vi "KPI.vi"(0 "Connection In":refnum<k7>, 5 "ID compresseur":dbl, 7 "Date Debut":timestamp format="%<%.0X %x>T", 9 "Date Fin":timestamp format="%<%.0X %x>T", 11 "Error in (no error)":errorcluster) -> (1 "Temps de fonctionnement total":string, 3 "Taux d’utilisation (%)":string, 4 "Connection Out":refnum<k7>, 6 "Pression moyenne":string, 10 "température moyenne":string, 12 "Nombre de démarrages / arrêts":string, 14 "Temps d'arret total":string, 15 "Error out":errorcluster)   [LabVIEW 2019]
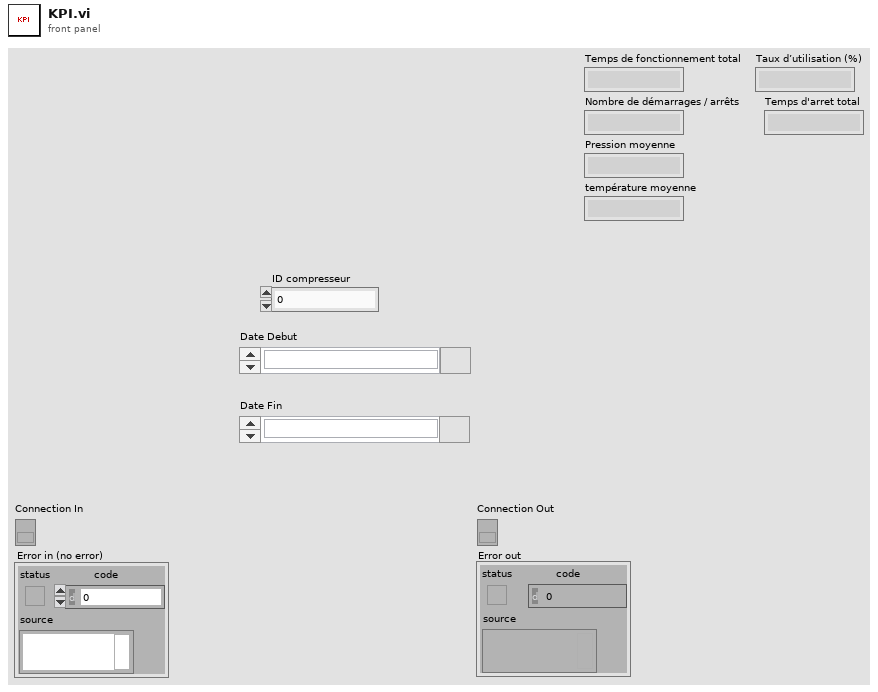
[diagram p1: front panel]
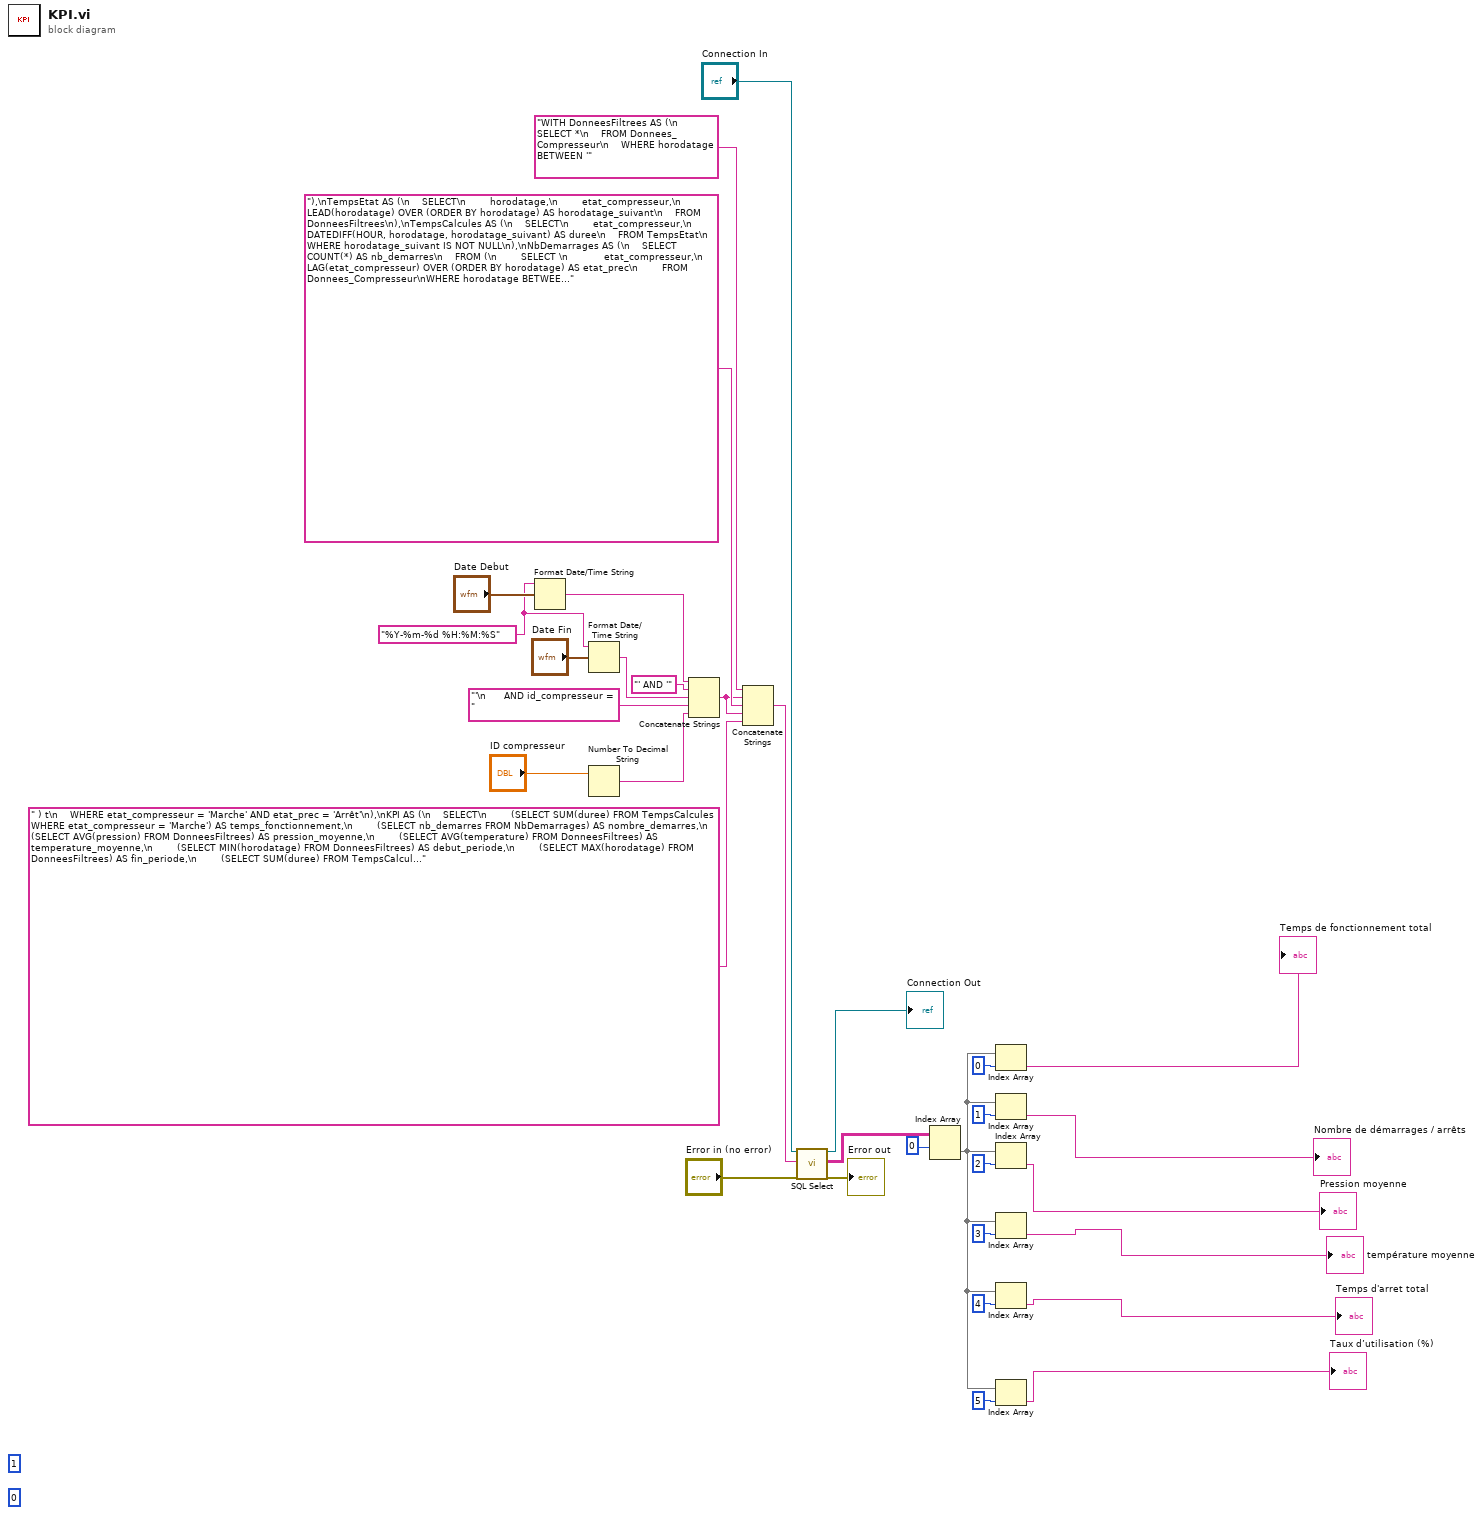
[diagram p0: block diagram]
diagram:
  (unwired) 0 ("index")
  (unwired) 1 ("index (row)")
  w29 = "%Y-%m-%d %H:%M:%S" ("time format string (%c)")
  n1 = Format Date/Time String(time format string (%c)=w29, seconds (now)="Date Debut") -> (date/time string=w25:string)  [unwired: 1 in]
  n2 = Format Date/Time String(time format string (%c)=w29, seconds (now)="Date Fin") -> (date/time string=w23:string)  [unwired: 1 in]
  n3 = Number To Decimal String(number="ID compresseur") -> (decimal integer string=w21:string)  [unwired: 1 in]
  n4 = Concatenate Strings(w25, "' AND '" ("string"), w23, "'\n      AND id_compresseur = " ("string"), w21) -> (w17:string)
  n5 = Concatenate Strings("WITH DonneesFiltrees AS (\n    SELECT *\n    FROM Donnees_Compresseur\n    WHERE horodatage BETWEEN '" ("string"), w17, "),\nTempsEtat AS (\n    SELECT\n        horodatage,\n        etat_compresseur,\n        LEAD(horodatage) OVER (ORDER BY horodatage) AS horodatage_suivant\n    FROM DonneesFiltrees\n),\nTempsCalcules AS (\n    SELECT\n        etat_compresseur,\n        DATEDIFF(HOUR, horodatage, horodatage_suivant) AS duree\n    FROM TempsEtat\n    WHERE horodatage_suivant IS NOT NULL\n),\nNbDemarrages AS (\n    SELECT COUNT(*) AS nb_demarres\n    FROM (\n        SELECT \n            etat_compresseur,\n            LAG(etat_compresseur) OVER (ORDER BY horodatage) AS etat_prec\n        FROM Donnees_Compresseur\nWHERE horodatage BETWEEN '" ("string"), w17, " ) t\n    WHERE etat_compresseur = 'Marche' AND etat_prec = 'Arrêt'\n),\nKPI AS (\n    SELECT\n        (SELECT SUM(duree) FROM TempsCalcules WHERE etat_compresseur = 'Marche') AS temps_fonctionnement,\n        (SELECT nb_demarres FROM NbDemarrages) AS nombre_demarres,\n        (SELECT AVG(pression) FROM DonneesFiltrees) AS pression_moyenne,\n        (SELECT AVG(temperature) FROM DonneesFiltrees) AS temperature_moyenne,\n        (SELECT MIN(horodatage) FROM DonneesFiltrees) AS debut_periode,\n        (SELECT MAX(horodatage) FROM DonneesFiltrees) AS fin_periode,\n        (SELECT SUM(duree) FROM TempsCalcules) AS duree_totale\n)\nSELECT\n    temps_fonctionnement AS [Temps de fonctionnement total (s)],\n    nombre_demarres AS [Nombre de démarrages / arrêts],\n    pression_moyenne AS [Pression moyenne],\n    temperature_moyenne AS [Température moyenne],\n    (duree_totale - temps_fonctionnement) AS [Temps d'arrêt total (s)],\n    ROUND(100.0 * temps_fonctionnement / NULLIF(DATEDIFF(HOUR, debut_periode, fin_periode), 0), 2) AS [Taux d'utilisation (%)]\nFROM KPI;" ("string")) -> (w14:string)
  n6 = call <vilib>:"SQL Select.vi"("Connection In"="Connection In", "SQL Query"=w14, "Error in (no error)"="Error in (no error)") -> ("Connection Out"=→"Connection Out":refnum<k7>, "Data"=w32:string[][], "Error out"=→"Error out":errorcluster)  [unwired: 14 in]
  n7 = Index Array(array=w32, index (row)=0 ("disabled index (col)")) -> (element=w13:string[])  [unwired: 1 in]
  n8 = Index Array(array=w13, index=0) -> (element=→"Temps de fonctionnement total":string)
  n9 = Index Array(array=w13, index=1) -> (element=→"Nombre de démarrages / arrêts":string)
  n10 = Index Array(array=w13, index=2) -> (element=→"Pression moyenne":string)
  n11 = Index Array(array=w13, index=3) -> (element=→"température moyenne":string)
  n12 = Index Array(array=w13, index=4) -> (element=→"Temps d'arret total":string)
  n13 = Index Array(array=w13, index=5) -> (element=→"Taux d’utilisation (%)":string)
